vi "dpd Complete.vi"(8 "error in (no error)":errorcluster, 10 "dpdStatus":i32, 11 "_hResourceContext":u32) -> (0 "error out":errorcluster, 1 "function return":bool, 2 "dpdStatus out":i32, 3 "_hResourceContext out":u32)   [LabVIEW 2013, in "QCAWLAN_DLL.lvlib"]
doc: "QCA_DLL_Export bool dpdComplete(HANDLE _hResourceContext, int* dpdStatus);"
uses:
  QCAWLAN_DLL.lvlib
  QCAWLAN_DLL.dll
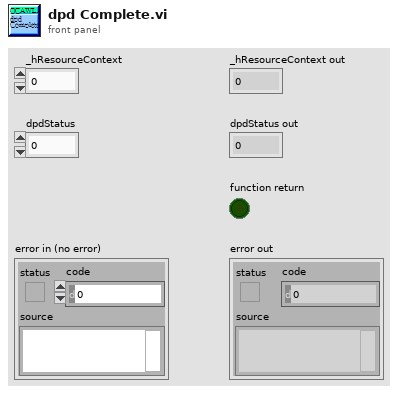
[diagram p1: front panel]
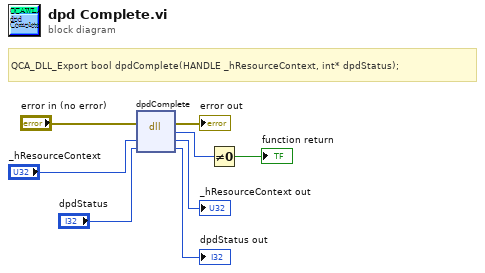
[diagram p0: block diagram]
diagram:
  # "QCA_DLL_Export bool dpdComplete(HANDLE _hResourceContext, int* dpdStatus);"
  n1 = dll-call lib="C:/Users/dave_yao/Desktop/Hitron/QCA9984 WLAN_LV2013/user.lib/QCAWLAN_DLL/QCAWLAN_DLL.*" fn="dpdComplete"(error in="error in (no error)", "_hResourceContext"="_hResourceContext", "dpdStatus"="dpdStatus") -> (error out=→"error out":errorcluster, w7:u8, "_hResourceContext"=→"_hResourceContext out":u32, "dpdStatus"=→"dpdStatus out":i32)  [unwired: 2 in, 1 out]
  n2 = Not Equal To 0?(x=w7) -> (x != 0?=→"function return":bool)
